vi "Flatten to String.vi"(8 "error in (no error)":errorcluster, 11 "TestLogValue in":refnum<class "TestLogValue.lvclass">) -> (0 "error out":errorcluster, 3 "Flattened Class":string)   [LabVIEW 2017, in "TestLogValue.lvclass"]
uses:
  TestLogValue.lvclass
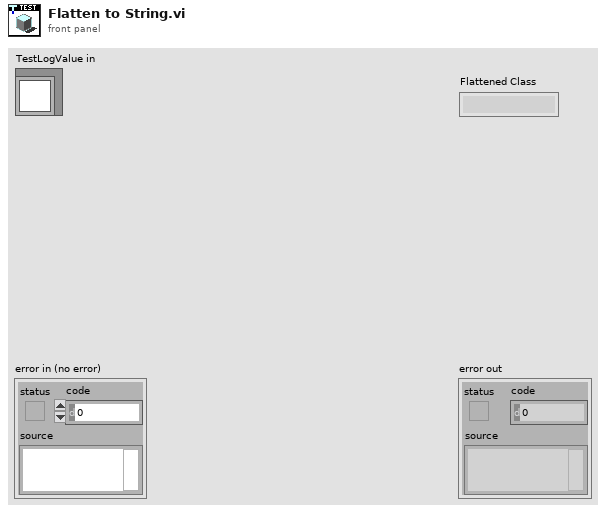
[diagram p1: front panel]
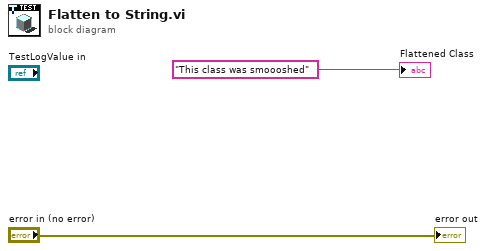
[diagram p0: block diagram]
diagram:
  "error out" <- "error in (no error)"
  "Flattened Class" <- "This class was smoooshed"
